vi "Debugging Page.vi"() -> ()   [LabVIEW 2024]
uses:
  <vilib>/Utility/miscctls.llb/LVRectTypeDef.ctl
panel:
  out "StringArr":string[](array[string])
  # "Made by Ramazan Burak Korkmaz"
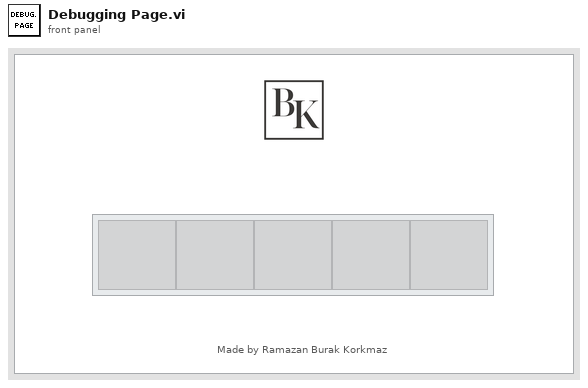
[diagram p1: front panel]
types:
  T1 = typedef "LVRectTypeDef.ctl" = cluster{"Left":i16, "Top":i16, "Right":i16, "Bottom":i16}
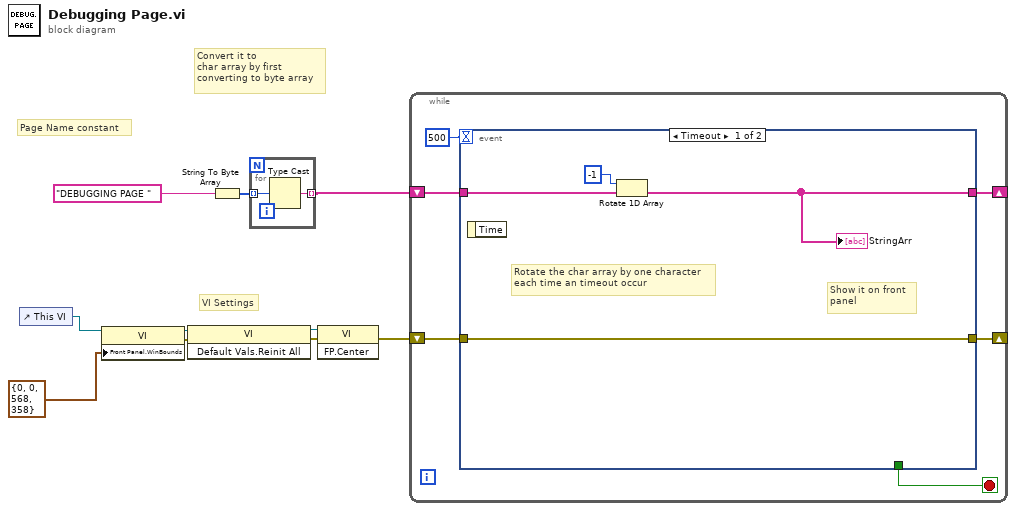
[diagram p0: block diagram]
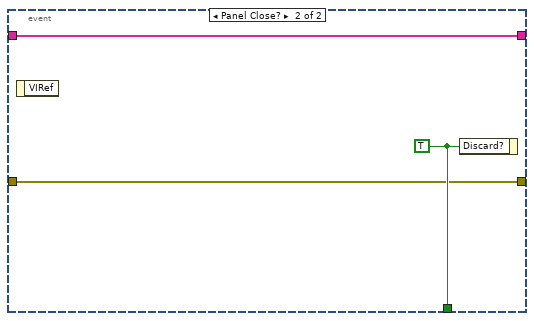
[diagram p2: hidden frame]
diagram:
  # "VI Settings"
  # "Convert it to\nchar array by first\nconverting to byte array"
  # "Page Name constant"
  n1 = control-ref of="This VI"() -> (w8:refnum<vi>)
  n2 = property class="VI"(reference=w8, "Front Panel.WinBounds"=T1 {"Left"=0, "Top"=0, "Right"=568, "Bottom"=358} ("Front Panel Window:Window Bounds")) -> (reference out=w10:refnum<vi>, error out=w9:errorcluster)  [unwired: 1 in]
  n3 = invoke class="VI" method="Default Vals.Reinit All"(reference=w10, error in=w9) -> (reference out=w7:refnum<vi>, error out=w6:errorcluster)  [unwired: 1 in, 1 out]
  n4 = String To Byte Array(string="DEBUGGING PAGE ") -> (unsigned byte array=w2:u8[])
  n5 = for {
    tunnel: w2 -> [w12] mode=indexing
    tunnel: [w11] -> w1 mode=indexing
    n6 = Type Cast(x=w12) -> (*(type *) &x=w11:string)  [unwired: 1 in]
  }
  n7 = invoke class="VI" method="FP.Center"(reference=w7, error in=w6) -> (error out=w4:errorcluster)  [unwired: 1 in, 2 out]
  n8 = while {
    shift-right: [w16] -> _
    shift-left: w1 -> [w17]
    shift-right: [w13] -> _
    shift-left: w4 -> [w14]
    stop <- w18 stop-if-true
    n9 = event shown="[0] Timeout" {
      selector: _ -> [_ _]
      dyn-events: _ -> [_ _]
      timeout: 500 -> [_ _]
      tunnel: [_ w25] -> w18
      tunnel: w17 -> [w22 w23]
      tunnel: [w21 w23] -> w16
      tunnel: w14 -> [w19 w24]
      tunnel: [w19 w24] -> w13
      event Timeout {
        # "Show it on front\npanel"
        # "Rotate the char array by one character\neach time an timeout occur"
        n10 = event-data() -> ()  [unwired: 1 in, 1 out]
        n11 = Rotate 1D Array(1:w22, 2:-1 ("n")) -> (0:w21:string[])
        "StringArr" <- w21
      }
      event Panel Close? {
        w25 = TRUE ("Discard?")
        n12 = event-data() -> ()  [unwired: 1 in, 1 out]
        n13 = event-data("Discard?"=w25) -> ()  [unwired: 1 in, 1 out]
      }
    }
  }
